vi "Send.vi"(8 "error in (no error)":errorcluster, 10 "Queue":refnum<class "Message Enqueuer.lvclass">, 11 "AcquireData in":refnum<class "AcquireData.lvclass">) -> (0 "error out":errorcluster, 3 "AcquireData out":refnum<class "AcquireData.lvclass">)   [LabVIEW 2011, in "AcquireData.lvclass"]
uses:
  AcquireData.lvclass
  <userlib>/_Frameworks/ActorFramework/Message Enqueuer/Message Enqueuer.lvclass
  <userlib>/_Frameworks/ActorFramework/Message Enqueuer/Message Enqueuer.lvclass/Message Enqueuer.ctl
  <userlib>/_Frameworks/ActorFramework/Message Priority Queue/Priority Enqueue.vi
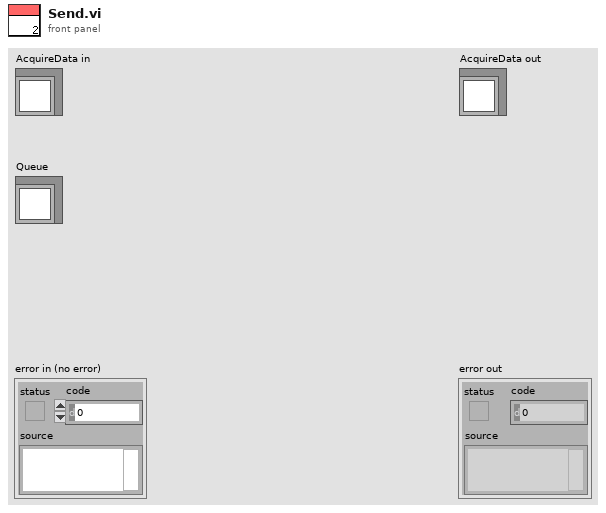
[diagram p1: front panel]
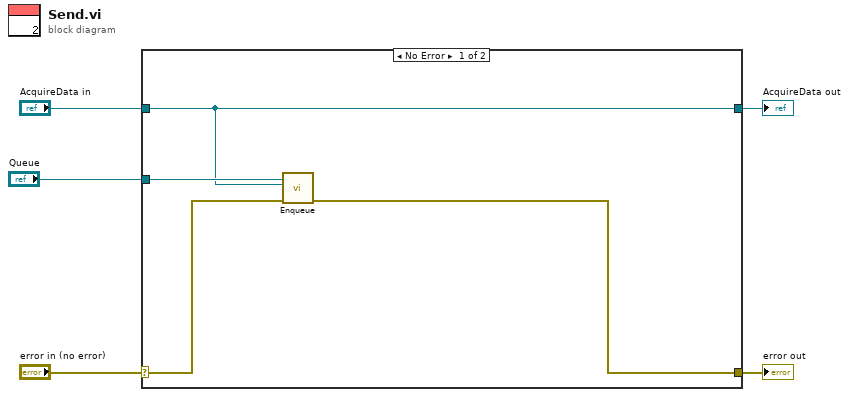
[diagram p0: block diagram]
diagram:
  n1 = case shown="No Error" "error in (no error)" {
    selector: "error in (no error)" -> [w7 w11]
    tunnel: [w6 w11] -> w4
    tunnel: [w8 w10] -> w2
    tunnel: "AcquireData in" -> [w8 w10]
    tunnel: "Queue" -> [w9 _]
    frame No Error {
      n2 = call <userlib>:"Enqueue.vi"("error in (no error)"=w7, "Message"=w8, "Message Enqueuer in"=w9) -> ("error out"=w6:errorcluster)  [unwired: 7 in, 1 out]
    }
    frame Error {
    }
  }
  "error out" <- w4
  "AcquireData out" <- w2
